vi "Write TR_SC_OD.vi"(8 "error in (no error)":errorcluster caption="entrée d'erreur (pas d'erreur)", 10 "TR_SC_OD":T1, 11 "Control-Client en entrée":refnum<class "Control-Client.lvclass">) -> (0 "error out":errorcluster caption="sortie d'erreur", 3 "Control-Client en sortie":refnum<class "Control-Client.lvclass">)   [LabVIEW 2018, in "Control-Client.lvclass"]
uses:
  Control-Client.lvclass
  dependecies/ControlsVIs/Clusters-def/graphs_TR.ctl
  Control-Client.lvclass/Control-Client.ctl
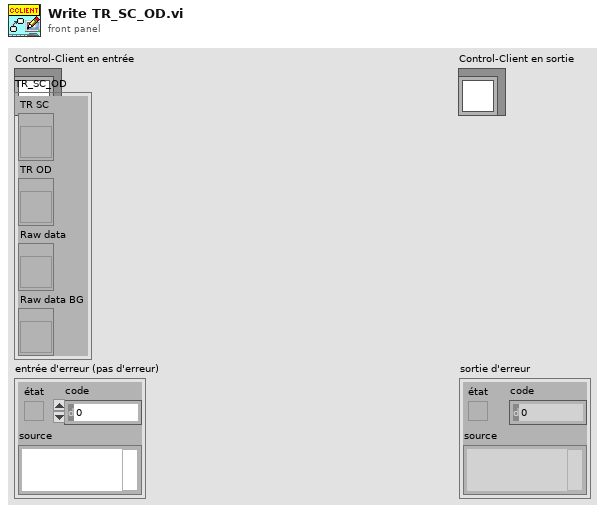
[diagram p1: front panel]
types:
  T1 = typedef "graphs_TR.ctl" = cluster{"TR SC":refnum<vi>, "TR OD":refnum<vi>, "Raw data":refnum<vi>, "Raw data BG":refnum<vi>}
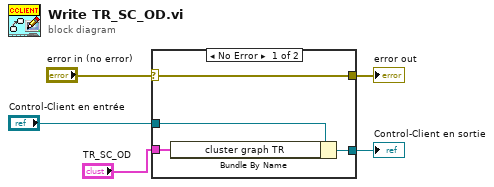
[diagram p0: block diagram]
diagram:
  n1 = case shown="No Error" "error in (no error)" {
    selector: "error in (no error)" -> [w9 w10]
    tunnel: [w9 w10] -> w4
    tunnel: [w7 w11] -> w2
    tunnel: "Control-Client en entrée" -> [w8 w11]
    tunnel: "TR_SC_OD" -> [w6 _]
    frame No Error {
      n2 = Bundle By Name(cluster=w8, "cluster graph TR"=w6) -> (w7:refnum<class "Control-Client.lvclass">)
    }
    frame Error {
    }
  }
  "error out" <- w4
  "Control-Client en sortie" <- w2
